vi "Auto_Global.vi"() -> ()   [LabVIEW 2015]
uses:
  Auto_Selection.ctl
panel:
  in  "Auto_Enable":bool
  in  "Auto_Selection":T1
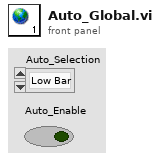
[diagram p1: front panel]
types:
  T1 = typedef "Auto_Selection.ctl" = enum16{"Low Bar", "Rough Terrain", "Rock Wall", "Ramparts", "Moat", "Cheval de Frise", "Portcullis", "None"}
diagram:
